vi "filename generator.vi"   [LabVIEW 2011, in "Filename Generator.lvlib"]
doc: "Generates a filename automatically. Choose the type from the pull-down menu."
uses:
  <instrlib>/Filename Generator.lvlib
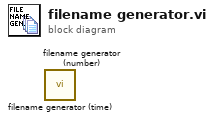
[diagram p0: block diagram]
diagram:
  n1 = call <instrlib>:"filename generator (time).vi"() -> ()  [unwired: 10 in, 2 out]
  n2 = call <instrlib>:"filename generator (number).vi"() -> ()  [unwired: 10 in, 2 out]
